vi "Measurement UI.vi"() -> ()   [LabVIEW 2021, in "PMIC UI.lvlib"]
uses:
  PMIC UI/PMIC UI.lvlib
  PMIC UI/State Data.ctl
  <vilib>/Utility/sysdir.llb/System Directory Type.ctl
  <vilib>/Utility/error.llb/DialogType.ctl
panel:
  in  "MeasGraphs":T1(tab)
  out "Error Message":string
  out "EfficiencyGraph":T2(graph)
  out "LoadRegulationGraph(V/A)":T2(graph)
  out "LoadRegulationGraph(%)":T2(graph)
  out "Load voltage deviation":dbl
  out "Load voltages":dbl
  out "Efficiency":dbl
  out "Load currents":dbl
  in  "Source Voltage":dbl=6.0 format="%#_6pV"
  in  "Load Current":dbl=5.0 format="%#_6pA"
  in  "Buffer graph":bool=TRUE
  in  "Load sense":i32(ring)=1009 caption="SENSE" items=["Local"=1008, "Remote"=1009]
  in  "Source sense":i32(ring)=1009 caption="SENSE" items=["Local"=1008, "Remote"=1009]
  out "Status":string
  in  "Load resource name":refnum<k15> caption="RESOURCE NAME"
  in  "Source resource name":refnum<k15> caption="RESOURCE NAME"
  in  "DUT setup time":dbl=1.0 caption="DUT SETUP TIME" format="%#_6ps"
  in  "Aperture time":dbl=0.005 caption="APERTURE TIME" format="%#_6ps"
  in  "Source delay":dbl=0.005 caption="SOURCE DELAY" format="%#_6ps"
  in  "Load voltage limit range":dbl=6.0 caption="VOLTAGE LIMIT RANGE" format="%#_6pV"
  in  "Source current limit":dbl=25.0 caption="CURRENT LIMIT" format="%#_6pA"
  in  "Source maximum power":dbl=140.0 caption="MAXIMUM POWER" format="%#_6pW"
  in  "Load configuration":string="Load configuration"
  in  "Source configuration":string="Source configuration"
  in  "Measurement settings":string="Measurement settings"
  in  "Nominal output voltage":dbl=3.3 caption="NOMINAL OUTPUT VOLTAGE" format="%#_6pV"
  in  "Mode of operation":T3(ring)=enum."Perform measurement" caption="MODE OF OPERATION"
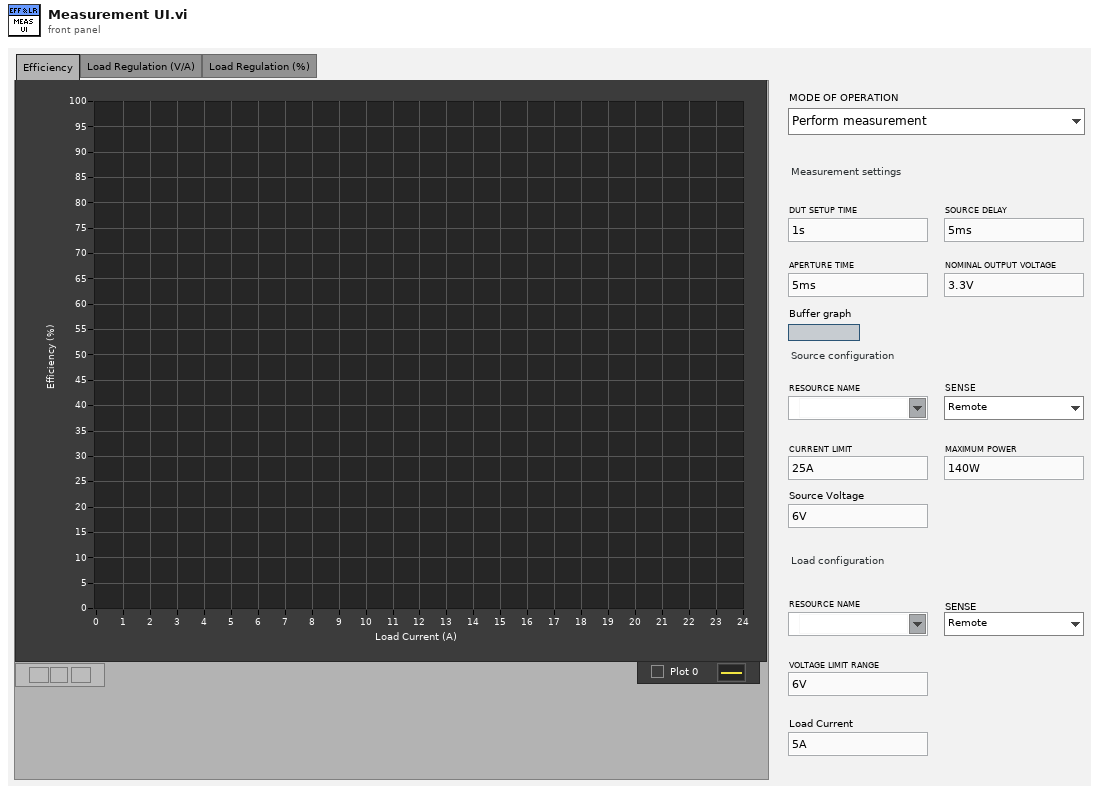
[diagram p1: front panel]
types:
  T1 = enum32{"Efficiency", "Load Regulation (V/A)", "Load Regulation (%)", "Hidden Controls"}
  T2 = cluster{"Load currents":dbl[], "Efficiency":dbl[]}[]
  T3 = enum32{"Power on the DUT", "Perform measurement", "Power off the DUT"}
  T4 = typedef "PMIC UI.lvlib/State Data.ctl" = cluster{"Source Voltage[]":dbl[], "Old Load Current":dbl, "EfficiencyGraph":cluster{"Load currents":dbl[], "Efficiency":dbl[]}[], "LoadGraph(V/A)":cluster{"Load currents":dbl[], "Efficiency":dbl[]}[], "LoadGraph(%)":cluster{"Load currents":dbl[], "Efficiency":dbl[]}[], "Execution Time":timestamp, "Debug file":path}
  T5 = typedef "System Directory Type.ctl" = i32
  T6 = typedef "DialogType.ctl" = u16
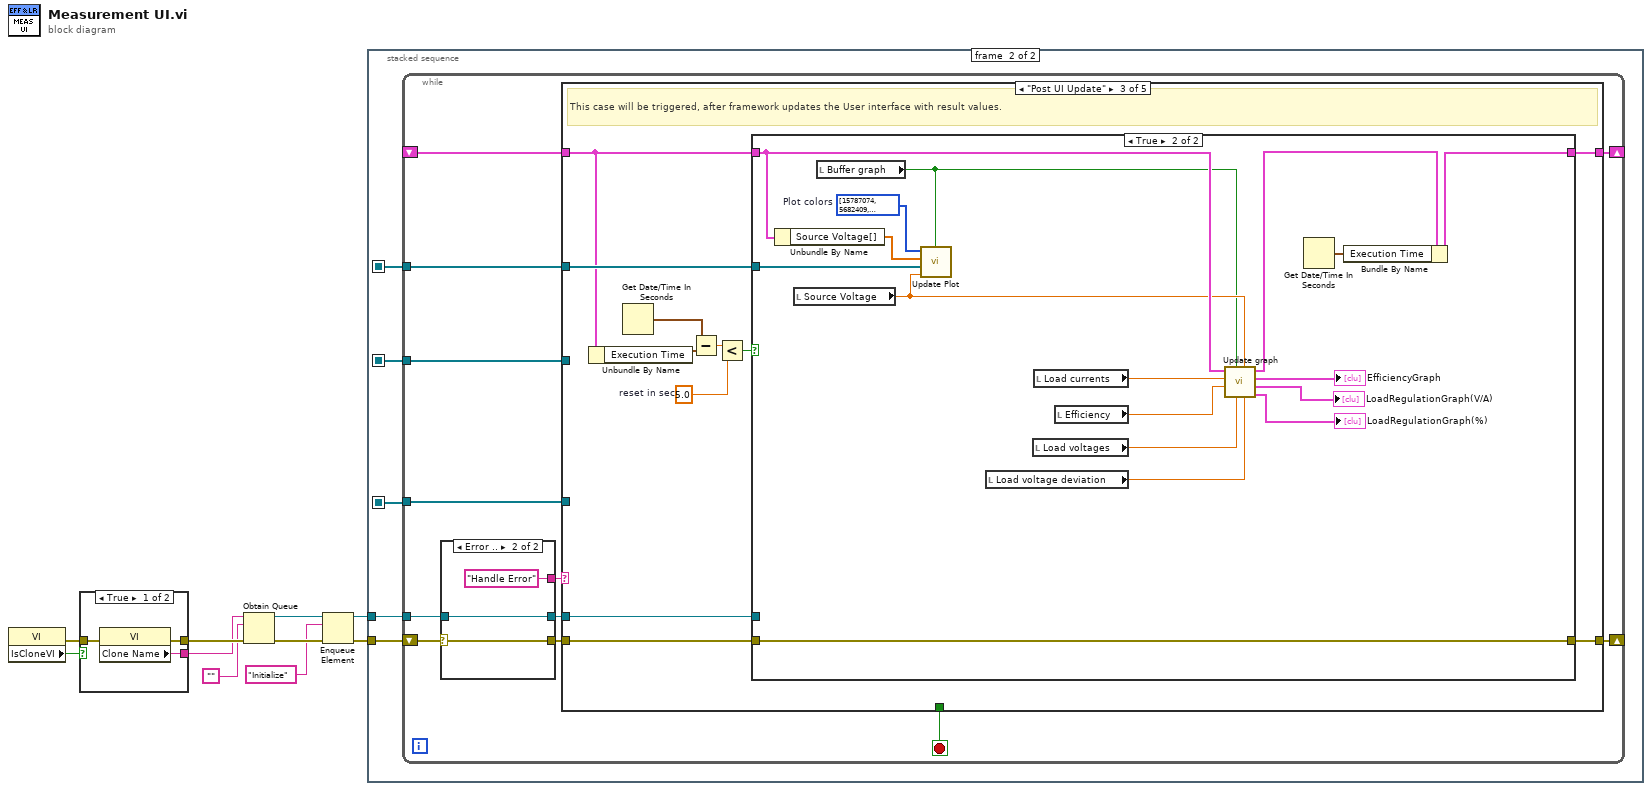
[diagram p0: block diagram]
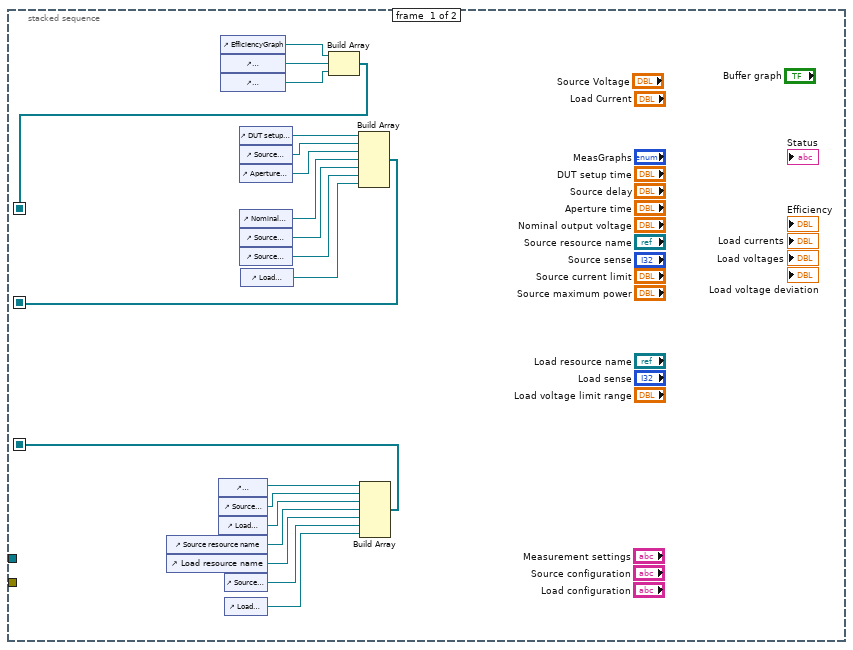
[diagram p2: hidden frame]
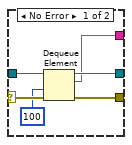
[diagram p3: hidden frame]
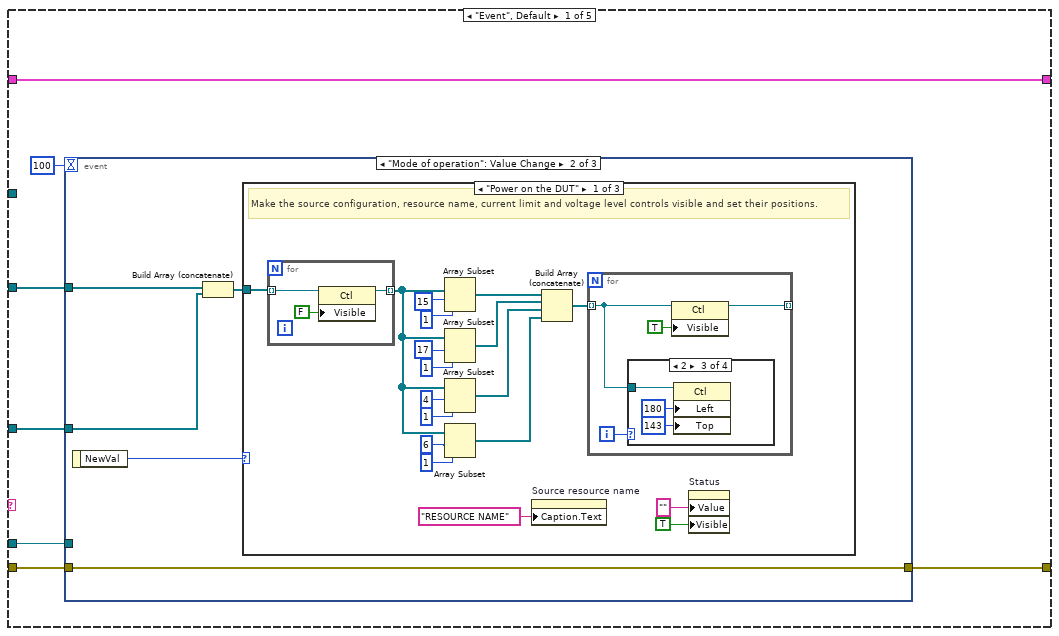
[diagram p4: hidden frame]
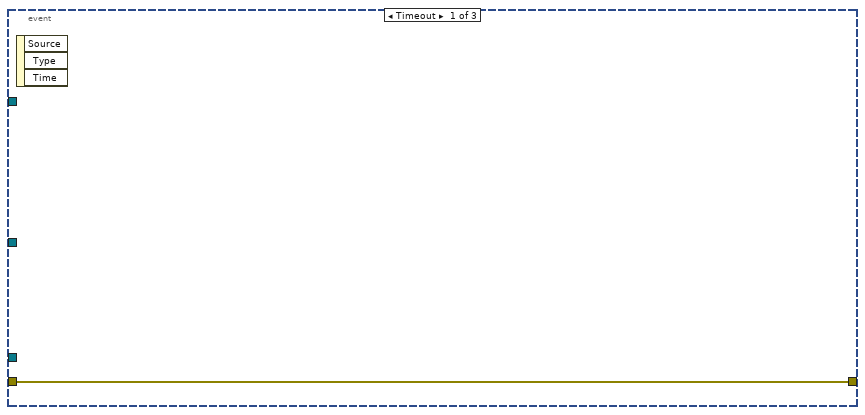
[diagram p5: hidden frame]
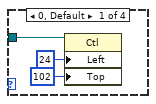
[diagram p6: hidden frame]
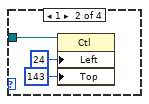
[diagram p7: hidden frame]
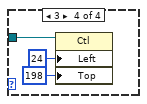
[diagram p8: hidden frame]
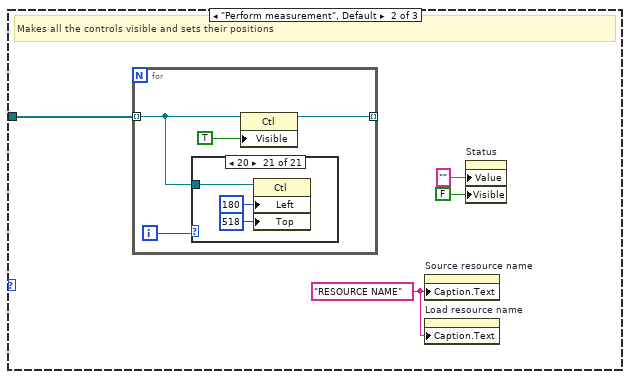
[diagram p9: hidden frame]
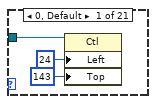
[diagram p10: hidden frame]
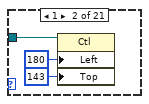
[diagram p11: hidden frame]
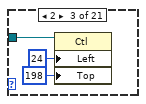
[diagram p12: hidden frame]
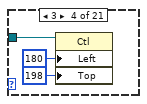
[diagram p13: hidden frame]
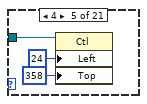
[diagram p14: hidden frame]
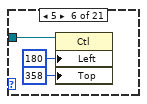
[diagram p15: hidden frame]
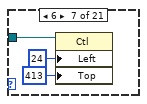
[diagram p16: hidden frame]
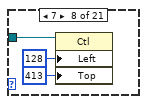
[diagram p17: hidden frame]
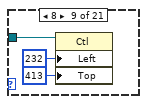
[diagram p18: hidden frame]
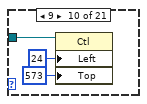
[diagram p19: hidden frame]
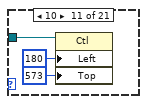
[diagram p20: hidden frame]
diagram:
  n1 = property class="VI"() -> (error out=w1:errorcluster, "IsCloneVI"=w2:bool)  [unwired: 2 in, 1 out]
  n2 = case shown="True" w2 {
    tunnel: [w13 w16] -> w10
    tunnel: [w12 w15] -> w9
    tunnel: w1 -> [w11 w14]
    frame True {
      n3 = property class="VI"(error in=w11) -> (error out=w13:errorcluster, "Clone Name"=w12:string)  [unwired: 1 in, 1 out]
    }
    frame False {
      n4 = property class="VI"(error in=w14) -> (error out=w16:errorcluster, "Name"=w15:string)  [unwired: 1 in, 1 out]
    }
  }
  n5 = Obtain Queue(name (unnamed)=w9, element data type="", error in (no error)=w10) -> (queue out=w6:refnum<queue>, error out=w8:errorcluster)  [unwired: 2 in, 1 out]
  n6 = Enqueue Element(queue=w6, element="Initialize", error in (no error)=w8) -> (queue out=w5:refnum<queue>, error out=w7:errorcluster)  [unwired: 1 in, 1 out]
  n7 = stacked-sequence {
    seq-local: [w19 _] -> [_ w39]
    seq-local: [w20 _] -> [_ w38]
    seq-local: [w21 _] -> [_ w37]
    tunnel: w7 -> [_ w41]
    tunnel: w5 -> [_ w40]
    frame #0 {
      n8 = control-ref of="Source resource name"() -> (w26:refnum<vi>)
      n9 = control-ref of="Load resource name"() -> (w25:refnum<vi>)
      n10 = control-ref of="Measurement settings"() -> (w29:refnum<vi>)
      n11 = control-ref of="Source configuration"() -> (w27:refnum<vi>)
      n12 = control-ref of="Load configuration"() -> (w28:refnum<vi>)
      n13 = control-ref of="EfficiencyGraph"() -> (w24:refnum<vi>)
      n14 = control-ref of="LoadRegulationGraph(V/A)"() -> (w23:refnum<vi>)
      n15 = control-ref of="LoadRegulationGraph(%)"() -> (w22:refnum<vi>)
      n16 = control-ref of="Source sense"() -> (w18:refnum<vi>)
      n17 = control-ref of="Load sense"() -> (w17:refnum<vi>)
      n18 = control-ref of="DUT setup time"() -> (w36:refnum<vi>)
      n19 = control-ref of="Source delay"() -> (w35:refnum<vi>)
      n20 = control-ref of="Aperture time"() -> (w34:refnum<vi>)
      n21 = control-ref of="Nominal output voltage"() -> (w30:refnum<vi>)
      n22 = control-ref of="Source current limit"() -> (w33:refnum<vi>)
      n23 = control-ref of="Source maximum power"() -> (w32:refnum<vi>)
      n24 = control-ref of="Load voltage limit range"() -> (w31:refnum<vi>)
      n25 = Build Array(w24, w23, w22) -> (w19:refnum<vi>[])
      n26 = Build Array(w36, w35, w34, w30, w33, w32, w31) -> (w20:refnum<vi>[])
      n27 = Build Array(w29, w27, w28, w26, w25, w18, w17) -> (w21:refnum<vi>[])
    }
    frame #1 {
      n28 = while {
        shift-right: [w48] -> _
        shift-left: w41 -> [w53]
        tunnel: w40 -> [w51]
        tunnel: w38 -> [w46]
        tunnel: w37 -> [w45]
        tunnel: w39 -> [w44]
        shift-right: [w43] -> _
        shift-left: _ -> [w42]
        stop <- w47 stop-if-true
        n29 = case shown="Error .." w53 {
          selector: w53 -> [w59 w62]
          tunnel: [w58 w62] -> w52
          tunnel: w51 -> [w57 w61]
          tunnel: [w56 w61] -> w50
          tunnel: [w55 "Handle Error"] -> w49
          frame No Error {
            n30 = Dequeue Element(queue=w57, timeout in ms (-1)=100, error in (no error)=w59) -> (queue out=w56:refnum<queue>, element=w55:string, error out=w58:errorcluster)  [unwired: 1 out]
          }
          frame Error {
          }
        }
        n31 = case shown="\"Post UI Update\"" w49 {
          tunnel: w52 -> [w68 w219 w230 w281 w285]
          tunnel: w50 -> [w66 _ w229 w279 _]
          tunnel: [w69 w213 w228 w273 w286] -> w48
          tunnel: [_ _ _ TRUE _] -> w47
          tunnel: w46 -> [w65 _ _ w271 _]
          tunnel: w45 -> [w64 _ _ w270 _]
          tunnel: w44 -> [_ w225 w238 w272 _]
          tunnel: [w63 w222 w237 w268 w287] -> w43
          tunnel: w42 -> [w63 _ w236 w268 w287]
          frame "Event", Default {
            n32 = event shown="[1] \"Mode of operation\": Value Change" {
              selector: _ -> [_ _ _]
              dyn-events: _ -> [_ _ _]
              timeout: 100 -> [_ _ _]
              tunnel: [w70 w71 w208] -> w69
              tunnel: w68 -> [w70 w71 w209]
              tunnel: w66 -> [_ _ w207]
              tunnel: w65 -> [_ w72 _]
              tunnel: w64 -> [_ w74 _]
              event Timeout {
                n33 = event-data() -> ()  [unwired: 1 in, 3 out]
              }
              event "Mode of operation": Value Change {
                n34 = event-data() -> ("NewVal"=w75:T3)  [unwired: 1 in]
                n35 = Build Array (concatenate)(w72, w74) -> (w73:refnum<vi>[])
                n36 = case shown="\"Power on the DUT\"" w75 {
                  tunnel: w73 -> [w85 w116 w189]
                  frame "Power on the DUT" {
                    # "Make the source configuration, resource name, current limit and voltage level controls visible and set their positions."
                    n37 = for {
                      tunnel: w85 -> [w96] mode=indexing
                      tunnel: [w94] -> w82 mode=indexing
                      n38 = property class="Ctl"(reference=w96, "Visible"=FALSE) -> (reference out=w94:refnum<vi>)  [unwired: 1 in, 1 out]
                    }
                    n39 = Array Subset(array=w82, index=15 ("length"), length=1 ("index")) -> (w84:refnum<vi>[])
                    n40 = Array Subset(array=w82, index=17 ("length"), length=1 ("index")) -> (w83:refnum<vi>[])
                    n41 = Array Subset(array=w82, index=4 ("length"), length=1 ("index")) -> (w81:refnum<vi>[])
                    n42 = Array Subset(array=w82, index=6 ("length"), length=1 ("index")) -> (w79:refnum<vi>[])
                    n43 = property on="Source resource name" class="IVIName"("Caption.Text"="RESOURCE NAME") -> ()  [unwired: 2 in, 2 out]
                    n44 = Build Array (concatenate)(w84, w83, w81, w79) -> (w80:refnum<vi>[])
                    n45 = for {
                      tunnel: [w99] -> _ mode=indexing
                      tunnel: w80 -> [w97] mode=indexing
                      i -> [w98]
                      n46 = case shown="2" w98 {
                        tunnel: w97 -> [w103 w106 w109 w112]
                        frame 0, Default {
                          n47 = property class="Ctl"(reference=w103, "Left"=24 ("Position:Left"), "Top"=102 ("Position:Top")) -> ()  [unwired: 1 in, 2 out]
                        }
                        frame 1 {
                          n48 = property class="Ctl"(reference=w106, "Left"=24 ("Position:Left"), "Top"=143 ("Position:Top")) -> ()  [unwired: 1 in, 2 out]
                        }
                        frame 2 {
                          n49 = property class="Ctl"(reference=w109, "Left"=180 ("Position:Left"), "Top"=143 ("Position:Top")) -> ()  [unwired: 1 in, 2 out]
                        }
                        frame 3 {
                          n50 = property class="Ctl"(reference=w112, "Left"=24 ("Position:Left"), "Top"=198 ("Position:Top")) -> ()  [unwired: 1 in, 2 out]
                        }
                      }
                      n51 = property class="Ctl"(reference=w97, "Visible"=TRUE) -> (reference out=w99:refnum<vi>)  [unwired: 1 in, 1 out]
                    }
                    n52 = property on="Status" class="Str"("Value"="" ("Status"), "Visible"=TRUE) -> ()  [unwired: 2 in, 2 out]
                  }
                  frame "Perform measurement", Default {
                    w115 = "RESOURCE NAME" ("Caption.Text")
                    # "Makes all the controls visible and sets their positions"
                    n53 = for {
                      tunnel: w116 -> [w117] mode=indexing
                      tunnel: [w119] -> _ mode=indexing
                      i -> [w118]
                      n54 = case shown="20" w118 {
                        tunnel: w117 -> [w123 w126 w129 w132 w135 w138 w141 w144 w147 w150 w153 w156 w159 w162 w165 w168 w171 w174 w177 w178 w181]
                        frame 0, Default {
                          n55 = property class="Ctl"(reference=w123, "Left"=24 ("Position:Left"), "Top"=143 ("Position:Top")) -> ()  [unwired: 1 in, 2 out]
                        }
                        frame 1 {
                          n56 = property class="Ctl"(reference=w126, "Left"=180 ("Position:Left"), "Top"=143 ("Position:Top")) -> ()  [unwired: 1 in, 2 out]
                        }
                        frame 2 {
                          n57 = property class="Ctl"(reference=w129, "Left"=24 ("Position:Left"), "Top"=198 ("Position:Top")) -> ()  [unwired: 1 in, 2 out]
                        }
                        frame 3 {
                          n58 = property class="Ctl"(reference=w132, "Left"=180 ("Position:Left"), "Top"=198 ("Position:Top")) -> ()  [unwired: 1 in, 2 out]
                        }
                        frame 4 {
                          n59 = property class="Ctl"(reference=w135, "Left"=24 ("Position:Left"), "Top"=358 ("Position:Top")) -> ()  [unwired: 1 in, 2 out]
                        }
                        frame 5 {
                          n60 = property class="Ctl"(reference=w138, "Left"=180 ("Position:Left"), "Top"=358 ("Position:Top")) -> ()  [unwired: 1 in, 2 out]
                        }
                        frame 6 {
                          n61 = property class="Ctl"(reference=w141, "Left"=24 ("Position:Left"), "Top"=413 ("Position:Top")) -> ()  [unwired: 1 in, 2 out]
                        }
                        frame 7 {
                          n62 = property class="Ctl"(reference=w144, "Left"=128 ("Position:Left"), "Top"=413 ("Position:Top")) -> ()  [unwired: 1 in, 2 out]
                        }
                        frame 8 {
                          n63 = property class="Ctl"(reference=w147, "Left"=232 ("Position:Left"), "Top"=413 ("Position:Top")) -> ()  [unwired: 1 in, 2 out]
                        }
                        frame 9 {
                          n64 = property class="Ctl"(reference=w150, "Left"=24 ("Position:Left"), "Top"=573 ("Position:Top")) -> ()  [unwired: 1 in, 2 out]
                        }
                        frame 10 {
                          n65 = property class="Ctl"(reference=w153, "Left"=180 ("Position:Left"), "Top"=573 ("Position:Top")) -> ()  [unwired: 1 in, 2 out]
                        }
                        frame 11 {
                          n66 = property class="Ctl"(reference=w156, "Left"=24 ("Position:Left"), "Top"=628 ("Position:Top")) -> ()  [unwired: 1 in, 2 out]
                        }
                        frame 12 {
                          n67 = property class="Ctl"(reference=w159, "Left"=128 ("Position:Left"), "Top"=628 ("Position:Top")) -> ()  [unwired: 1 in, 2 out]
                        }
                        frame 13 {
                          n68 = property class="Ctl"(reference=w162, "Left"=232 ("Position:Left"), "Top"=628 ("Position:Top")) -> ()  [unwired: 1 in, 2 out]
                        }
                        frame 14 {
                          n69 = property class="Ctl"(reference=w165, "Left"=24 ("Position:Left"), "Top"=102 ("Position:Top")) -> ()  [unwired: 1 in, 2 out]
                        }
                        frame 15 {
                          n70 = property class="Ctl"(reference=w168, "Left"=24 ("Position:Left"), "Top"=262 ("Position:Top")) -> ()  [unwired: 1 in, 2 out]
                        }
                        frame 16 {
                          n71 = property class="Ctl"(reference=w171, "Left"=24 ("Position:Left"), "Top"=477 ("Position:Top")) -> ()  [unwired: 1 in, 2 out]
                        }
                        frame 17 {
                          n72 = property class="Ctl"(reference=w174, "Left"=24 ("Position:Left"), "Top"=303 ("Position:Top")) -> ()  [unwired: 1 in, 2 out]
                        }
                        frame 18 {
                          n73 = property class="Ctl"(reference=w177, "Left"=24 ("Position:Left"), "Top"=518 ("Position:Top")) -> ()  [unwired: 1 in, 2 out]
                        }
                        frame 19 {
                          n74 = property class="Ctl"(reference=w178, "Left"=180 ("Position:Left"), "Top"=303 ("Position:Top")) -> ()  [unwired: 1 in, 2 out]
                        }
                        frame 20 {
                          n75 = property class="Ctl"(reference=w181, "Left"=180 ("Position:Left"), "Top"=518 ("Position:Top")) -> ()  [unwired: 1 in, 2 out]
                        }
                      }
                      n76 = property class="Ctl"(reference=w117, "Visible"=TRUE) -> (reference out=w119:refnum<vi>)  [unwired: 1 in, 1 out]
                    }
                    n77 = property on="Source resource name" class="IVIName"("Caption.Text"=w115) -> ()  [unwired: 2 in, 2 out]
                    n78 = property on="Load resource name" class="IVIName"("Caption.Text"=w115) -> ()  [unwired: 2 in, 2 out]
                    n79 = property on="Status" class="Str"("Value"="" ("Status"), "Visible"=FALSE) -> ()  [unwired: 2 in, 2 out]
                  }
                  frame "Power off the DUT" {
                    # "Makes only the Source and Load Resource Name controls visible and sets their positions"
                    n80 = for {
                      tunnel: w189 -> [w194] mode=indexing
                      tunnel: [w193] -> w188 mode=indexing
                      n81 = property class="Ctl"(reference=w194, "Visible"=FALSE) -> (reference out=w193:refnum<vi>)  [unwired: 1 in, 1 out]
                    }
                    n82 = Array Subset(array=w188, index=17 ("length"), length=2 ("index")) -> (w190:refnum<vi>[])
                    n83 = property on="Source resource name" class="IVIName"("Caption.Text"="SOURCE RESOURCE NAME") -> ()  [unwired: 2 in, 2 out]
                    n84 = property on="Load resource name" class="IVIName"("Caption.Text"="LOAD RESOURCE NAME") -> ()  [unwired: 2 in, 2 out]
                    n85 = for {
                      tunnel: w190 -> [w196] mode=indexing
                      tunnel: [w198] -> _ mode=indexing
                      i -> [w197]
                      n86 = case shown="0, Default" w197 {
                        tunnel: w196 -> [w202 w205]
                        frame 0, Default {
                          n87 = property class="Ctl"(reference=w202, "Left"=24 ("Position:Left"), "Top"=102 ("Position:Top")) -> ()  [unwired: 1 in, 2 out]
                        }
                        frame 1 {
                          n88 = property class="Ctl"(reference=w205, "Left"=24 ("Position:Left"), "Top"=157 ("Position:Top")) -> ()  [unwired: 1 in, 2 out]
                        }
                      }
                      n89 = property class="Ctl"(reference=w196, "Visible"=TRUE) -> (reference out=w198:refnum<vi>)  [unwired: 1 in, 1 out]
                    }
                    n90 = property on="Status" class="Str"("Value"="" ("Status"), "Visible"=TRUE) -> ()  [unwired: 2 in, 2 out]
                  }
                }
              }
              event Panel Close? {
                n91 = event-data() -> ()  [unwired: 1 in, 4 out]
                n92 = Enqueue Element(queue=w207, element="Exit", error in (no error)=w209) -> (error out=w208:errorcluster)  [unwired: 1 in, 2 out]
                n93 = event-data("Discard?"=TRUE) -> ()  [unwired: 1 in, 1 out]
              }
            }
          }
          frame "Initialize" {
            w218 = T5 2 items=["User Home"=0, "User Desktop"=1, "User Documents"=2, "User Application Data"=3, "User Preferences"=4, "User Temporary"=5, "Public Documents"=6, "Public Application Data"=7, "Public Preferences"=8, "Public Cache"=13, "System Core Libraries"=9, "System Installed Libraries"=10, "Application Files"=11, "Boot Volume Root"=12] ("system directory type")
            n94 = for {
              tunnel: w225 -> [w226] mode=indexing
              n95 = property class="XYGraph (strict)"(reference=w226, "ActPaletteTool"=2 ("Palette:Active Tool")) -> ()  [unwired: 1 in, 2 out]
            }
            n96 = property on="Buffer graph" class="Bool (strict)"("Visible"=TRUE) -> ()  [unwired: 2 in, 2 out]
            n97 = property on="Status" class="Str"("Visible"=FALSE) -> ()  [unwired: 2 in, 2 out]
            n98 = call <vilib>:"Get System Directory.vi"("system directory type"=w218) -> ("system directory"=w217:path)  [unwired: 10 in]
            n99 = Build Path(base path=w217, name or relative path=path "InstrumentStudio Projects/Effieciency Graph.csv") -> (appended path=w214:path)
            n100 = call <vilib>:"Create File with Incrementing Suffix.vi"("error in (no error)"=w219, "file path"=w214) -> ("error out"=w215:errorcluster, "actual path"=w211:path, "refnum out"=w212:refnum<file>)  [unwired: 7 in]
            n101 = Get Date/Time In Seconds() -> (seconds since 1Jan1904=w220:timestamp)
            n102 = Bundle By Name(cluster=T4 {"Source Voltage[]"=[], "Old Load Current"=0.0, "EfficiencyGraph"=[], "LoadGraph(V/A)"=[], "LoadGraph(%)"=[], "Execution Time"=timestamp(0 s since 1904-01-01), "Debug file"=path ""} ("UI"), "Execution Time"=w220, "Debug file"=w211) -> (w222:T4)
            n103 = Close File(refnum=w212, error in=w215) -> (error out=w213:errorcluster)  [unwired: 1 out]
          }
          frame "Post UI Update" {
            w232 = 5.0  # reset in sec
            # "This case will be triggered, after framework updates the User interface with result values."
            n104 = Unbundle By Name(w236) -> ("Execution Time"=w234:timestamp)
            n105 = Get Date/Time In Seconds() -> (seconds since 1Jan1904=w235:timestamp)
            n106 = Subtract(x=w235, y=w234) -> (x-y=w233:dbl)
            n107 = Less?(x=w233, y=w232) -> (x < y?=w231:bool)
            n108 = case shown="True" w231 {
              tunnel: w238 -> [_ w267]
              tunnel: w236 -> [w241 w253]
              tunnel: [w240 w256] -> w237
              tunnel: w230 -> [w244 w257]
              tunnel: w229 -> [w243 _]
              tunnel: [w242 w257] -> w228
              frame False {
                # "Assuming that the user will take atleast 5 seconds for next sequence run.\nThe 5 seconds value chosed because measurement always took more than\n5 seconds to execute."
                n109 = disable-structure shown="Enabled" {
                  disable-tunnel: w244 -> [w249 w250]
                  disable-tunnel: w243 -> [w248 _]
                  disable-tunnel: [w245 w250] -> w242
                  frame Enabled {
                    n110 = Enqueue Element(queue=w248, element="Initialize", timeout in ms (-1)=100, error in (no error)=w249) -> (error out=w245:errorcluster)  [unwired: 2 out]
                  }
                  frame Disabled {
                  }
                }
                n111 = Get Date/Time In Seconds() -> (seconds since 1Jan1904=w239:timestamp)
                n112 = Bundle By Name(cluster=w241, "Execution Time"=w239) -> (w240:T4)
              }
              frame True {
                w258 = u32[] [15787074, 5682409, 15535092, 40563, 13983232, 35009, 15113984, 13400487, 15993633, 10221451, 8148942, 15869817, 32914, 10196480, 6271923, 16355671]  # Plot colors
                n113 = Unbundle By Name(w253) -> ("Source Voltage[]"=w262:dbl[])
                n114 = local read "Source Voltage"() -> (w252:dbl)
                n115 = local read "Buffer graph"() -> (w251:bool)
                n116 = call "Update Plot.vi"("Buffer"=w251, "Source Voltage"=w252, "XY Graphs"=w267, "Source Voltage[]"=w262, "Plot colors"=w258) -> ()  [unwired: 7 in]
                n117 = local read "Load voltage deviation"() -> (w263:dbl)
                n118 = local read "Load voltages"() -> (w264:dbl)
                n119 = local read "Load currents"() -> (w266:dbl)
                n120 = local read "Efficiency"() -> (w265:dbl)
                n121 = call "Update graph.vi"("Load voltage deviation"=w263, "Source Voltage"=w252, "Load voltages"=w264, "Buffer graph"=w251, "Efficiency"=w265, "Load currents"=w266, "UI in"=w253) -> ("LoadGraph(%)"=→"LoadRegulationGraph(%)":T2, "LoadGraph(V/A)"=→"LoadRegulationGraph(V/A)":T2, "EfficiencyGraph"=→"EfficiencyGraph":T2, "UI out"=w261:T4)  [unwired: 1 in]
                n122 = Get Date/Time In Seconds() -> (seconds since 1Jan1904=w255:timestamp)
                n123 = Bundle By Name(cluster=w261, "Execution Time"=w255) -> (w256:T4)
              }
            }
          }
          frame "Exit" {
            # "This case is triggered to close the User Interface from framework"
            n124 = Flush Queue(queue=w279, error in (no error)=w281) -> (queue out=w278:refnum<queue>, error out=w277:errorcluster)  [unwired: 1 out]
            n125 = Release Queue(queue=w278, force destroy? (F)=TRUE, error in (no error)=w277) -> (error out=w274:errorcluster)  [unwired: 2 out]
            n126 = Build Array (concatenate)(w272, w271, w270) -> (w269:refnum<vi>[])
            n127 = Close Reference(reference=w269) -> (error out=w275:errorcluster)  [unwired: 1 in]
            n128 = Merge Errors(w275, w274) -> (w273:errorcluster)
          }
          frame "Handle Error" {
            w283 = T6 0 items=["no dialog", "OK message", "continue or stop message", "OK message + warnings", "continue/stop + warnings"] ("type of dialog (OK msg:1)")
            n129 = call <vilib>:"Simple Error Handler.vi"("type of dialog (OK msg:1)"=w283, "error in (no error)"=w285) -> ("error out"=w284:errorcluster, "message"=→"Error Message":string)  [unwired: 3 in, 3 out]
            n130 = call <vilib>:"Clear Errors.vi"("error in (no error)"=w284) -> ("error out"=w286:errorcluster)  [unwired: 5 in, 1 out]
          }
        }
      }
    }
  }
